vi "gyro_simple_display.vi"(0 "waveform":waveform(dbl), 1 "threshold":dbl=0.4 format="%0.2f", 2 "width [Hz]":dbl=20.0, 3 "felharmonikus N":i32, 4 "width":i32=3 min=3, 5 "crossing level":dbl=-0.15, 7 "end":dbl=1.0) -> (14 "mean of peaks":dbl format="%0.2f", 15 "standard deviation of peaks":dbl format="%0.2f", 16 "Impulse Integral":dbl[](array[numeric]), 17 "stroke rate":dbl[](array[numeric]), 18 "Csapásszám [stroke/min]":dbl, 19 "SNR":dbl)   [LabVIEW 2017]
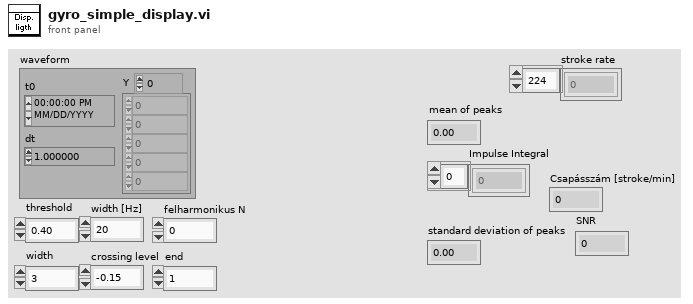
[diagram p1: front panel]
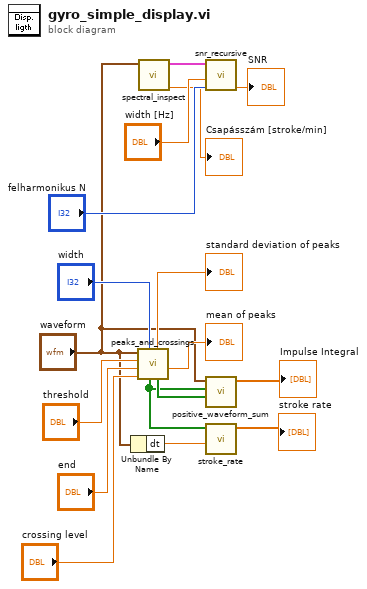
[diagram p0: block diagram]
diagram:
  n1 = Unbundle By Name("waveform") -> ("dt"=w6:dbl)
  n2 = call "peaks_and_crossings.vi"("width"="width", "crossing level"="crossing level", "end"="end", "threshold"="threshold", "waveform"="waveform") -> ("mean of peaks"=→"mean of peaks":dbl, "plus-minus"=w16:bool[], "standard deviation of peaks"=→"standard deviation of peaks":dbl, "minus-plus"=w15:bool[])  [unwired: 3 out]
  n3 = call "spectral_inspect.vi"("waveform"="waveform") -> ("Csapásszám [stroke/min]"=→"Csapásszám [stroke/min]":dbl, "PSD"=w17:cluster{"f0":dbl, "df":dbl, "magnitude":dbl[]})  [unwired: 7 in, 2 out]
  n4 = call "snr_recursive.vi"("felharmonikus N"="felharmonikus N", "width [Hz]"="width [Hz]", "PSD"=w17) -> ("SNR"=→"SNR":dbl)  [unwired: 5 in, 3 out]
  n5 = call "positive_waveform_sum.vi"("plus-minus"=w16, 10:w15, "waveform"="waveform") -> ("Integral X"=→"Impulse Integral":dbl[])  [unwired: 7 in, 1 out]
  n6 = call "stroke_rate.vi"("dt"=w6, "minus-plus"=w15) -> ("stroke rate"=→"stroke rate":dbl[])  [unwired: 9 in]
